vi "Display Sel Image.vi"(8 "error in":errorcluster, 9 "Img Indicator":refnum<vi>, 10 "Selected Image":string, 11 "Controller in":refnum<class "Controller.lvclass">) -> (0 "error out":errorcluster, 3 "Controller out":refnum<class "Controller.lvclass">)   [LabVIEW 2021, in "Controller.lvlib" / "Controller.lvclass"]
uses:
  Controller.lvclass
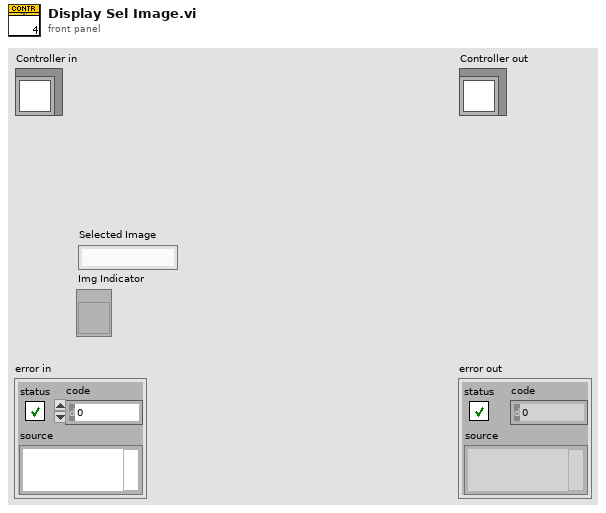
[diagram p1: front panel]
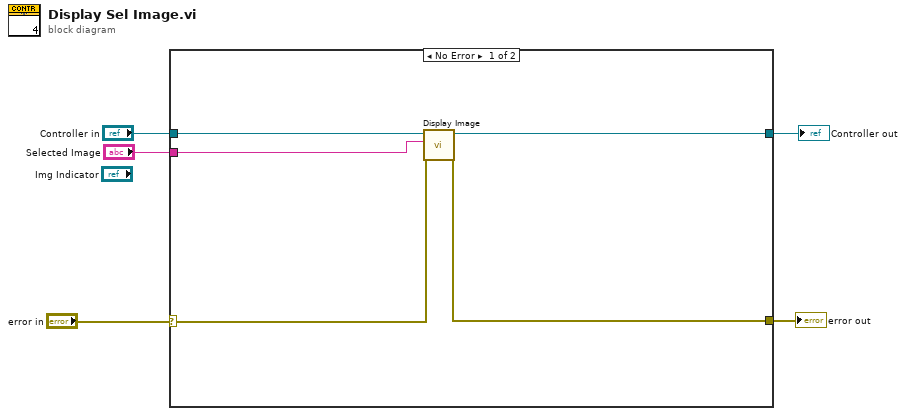
[diagram p0: block diagram]
diagram:
  n1 = case shown="No Error" "error in" {
    selector: "error in" -> [w8 w11]
    tunnel: "Controller in" -> [w9 w12]
    tunnel: [w10 w12] -> w4
    tunnel: [w7 w11] -> w2
    tunnel: "Selected Image" -> [w6 _]
    frame No Error {
      n2 = call-dynamic "Display Image.vi"("error in (no error)"=w8, "File Name"=w6, "Controller in"=w9) -> ("error out"=w7:errorcluster, "Controller out"=w10:refnum<class "Controller.lvclass">)  [unwired: 7 in]
    }
    frame Error {
    }
  }
  "error out" <- w2
  "Controller out" <- w4
